vi "set channel property.vi"(8 "error in":errorcluster, 9 "Value":variant, 10 "Property":T2, 11 "Card.Channel":T1={" Card.Channel"=1.12, "Crate"=0} {"Card.Channel" format="%.2f"}) -> (0 "error out":errorcluster, 1 "Value Out":variant, 2 "Property Out":T2, 3 "Card.Channel Out":T1={" Card.Channel"=1.12, "Crate"=0} {"Card.Channel" format="%.2f"})   [LabVIEW 2018]
uses:
  channel.ctl
  Channel Properties.ctl
panel:
  out "VISA out":refnum<visa-resource-name>
  in  "VISA in":refnum<visa-resource-name>
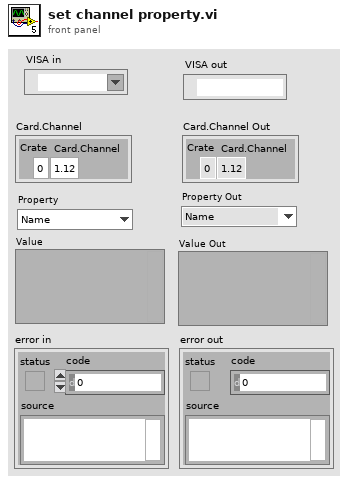
[diagram p1: front panel]
types:
  T1 = typedef "channel.ctl" = cluster{" Card.Channel":dbl, "Crate":i32}
  T2 = typedef "Channel Properties.ctl" = enum16{"Name", "Vset", "Vfile", "Vswmax", "Iset", "Enable", "Flag", "Vbackup"}
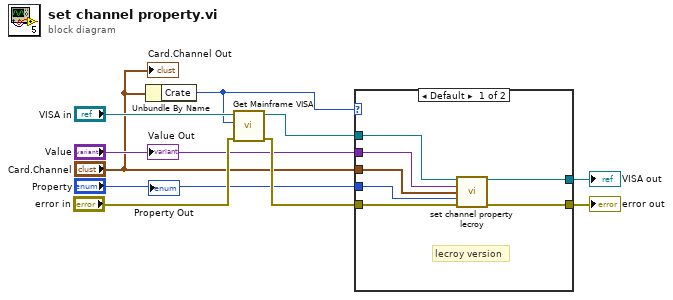
[diagram p0: block diagram]
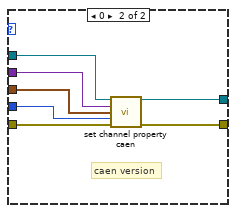
[diagram p2: hidden frame]
diagram:
  n1 = Unbundle By Name("Card.Channel") -> ("Crate"=w4:i32)
  n2 = call "Get Mainframe VISA.vi"("Error In"="error in", "Crate"=w4, "VISA In"="VISA in") -> ("Error Out"=w7:errorcluster, "VISA out"=w5:refnum<visa-resource-name>)  [unwired: 6 in, 1 out]
  n3 = case shown="Default" w4 {
    tunnel: w5 -> [w11 w24]
    tunnel: "Value" -> [w14 w23]
    tunnel: "Card.Channel" -> [w13 w22]
    tunnel: "Property" -> [w12 w21]
    tunnel: w7 -> [w15 w20]
    tunnel: [w17 w19] -> w10
    tunnel: [w16 w18] -> w9
    frame Default {
      # "lecroy version"
      n4 = call "set channel property lecroy.vi"("VISA in"=w11, "Value"=w14, "Channel"=w13, "Property"=w12, "error in"=w15) -> ("VISA out"=w17:refnum<visa-resource-name>, "error out"=w16:errorcluster)  [unwired: 9 in]
    }
    frame 0 {
      # "caen version"
      n5 = call "set channel property caen.vi"("VISA in"=w24, "Value"=w23, "Channel"=w22, "Property"=w21, "error in"=w20) -> ("VISA out"=w19:refnum<visa-resource-name>, "error out"=w18:errorcluster)  [unwired: 9 in]
    }
  }
  "VISA out" <- w10
  "error out" <- w9
  "Property Out" <- "Property"
  "Value Out" <- "Value"
  "Card.Channel Out" <- "Card.Channel"
